vi "pb_outp.vi"(1 "error in (no error)":errorcluster, 2 "8-bit data":u8, 3 "8-bit address offset":u8) -> (0 "error out":errorcluster)   [LabVIEW 2013, in "PulseBlaster.lvlib"]
uses:
  PulseBlaster.lvlib
  spinapi.dll
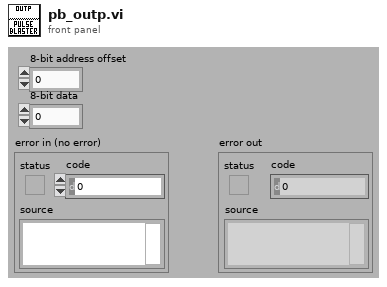
[diagram p1: front panel]
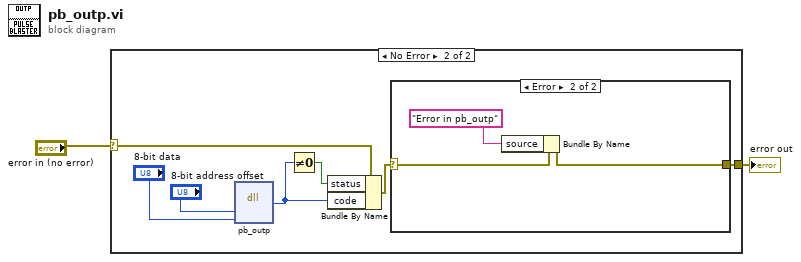
[diagram p0: block diagram]
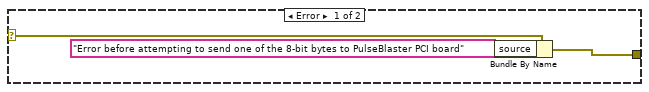
[diagram p2: hidden frame]
diagram:
  n1 = case shown="No Error" "error in (no error)" {
    selector: "error in (no error)" -> [w5 w10]
    tunnel: [w4 w8] -> w1
    frame Error {
      n2 = Bundle By Name(cluster=w5, "source"="Error before attempting to send one of the 8-bit bytes to PulseBlaster PCI board") -> (w4:errorcluster)
    }
    frame No Error {
      n3 = dll-call lib="C:/Users/cherold/Documents/SVNrepo_local/branches/TableTest_Auto/codes/DeviceVIs/Pulseblaster/spinapi.dll" fn="pb_outp"("address"="8-bit address offset", "data"="8-bit data") -> ("return type"=w11:i32)  [unwired: 5 in, 2 out]
      n4 = Not Equal To 0?(x=w11) -> (x != 0?=w12:bool)
      n5 = Bundle By Name(cluster=w10, "status"=w12, "code"=w11) -> (w9:errorcluster)
      n6 = case shown="Error" w9 {
        selector: w9 -> [w13 w15]
        tunnel: [w13 w14] -> w8
        frame No Error {
        }
        frame Error {
          n7 = Bundle By Name(cluster=w15, "source"="Error in pb_outp") -> (w14:errorcluster)
        }
      }
    }
  }
  "error out" <- w1
